vi "Post Tolerance edit.vi"(8 "error in (no error)":errorcluster, 10 "Coords":T1, 11 "ZenGage v3.0 UI in":refnum<class "ZenGage v3.0 UI.lvclass">) -> (0 "error out":errorcluster, 3 "ZenGage v3.0 UI out":refnum<class "ZenGage v3.0 UI.lvclass">)   [LabVIEW 2015, in "ZenGage v3.0 UI.lvclass"]
uses:
  ZenGage v3.0 UI.lvclass
  <vilib>/Utility/miscctls.llb/LVPoint32TypeDef.ctl
  ZenGage v3.0 UI.lvclass/ZenGage v3.0 UI.ctl
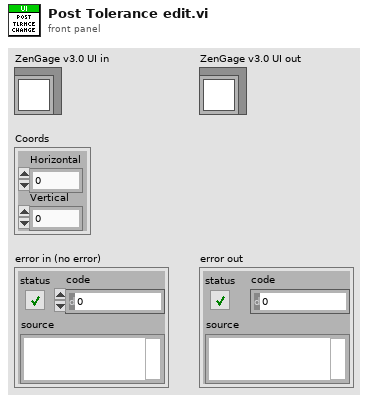
[diagram p1: front panel]
types:
  T1 = typedef "LVPoint32TypeDef.ctl" = cluster{"Horizontal":i32, "Vertical":i32}
  T2 = typedef "ZenGage v3.0 UI.lvclass/Edit Tolerance Input.ctl" = cluster{"ETL controls":T3, "Input Data Cluster":cluster{"Measurement Values":string[][], "Cluster of Limits":cluster{"LSL":dbl, "USL":dbl, "LCL":dbl, "UCL":dbl}, "Rack Selection":T4, "M and N Array":cluster{"M1":u64, "M2":u64, "N1":u64, "N2":u64}[], "Ticked Measurement Index":u32[], "Measurements Enabled":bool[], "Current Active Position":T1, "Current ticked measurement":dbl}}
  T3 = typedef "ETL controls.ctl" = cluster{"Measurement\n ListBox":refnum<vi>, "Cluster of limits":refnum<vi>, "Thresholds limits":refnum<vi>, "Bias Correction":refnum<vi>, "Linearity Correction":refnum<vi>}
  T4 = typedef "ZenGage v3.0 UI.lvclass/Rack Selection.ctl" = enum16{"Both Racks", "Rack 2", "Rack 1"}
  T5 = enum8{"Enabled", "Disabled", "Disabled and Grayed Out"}
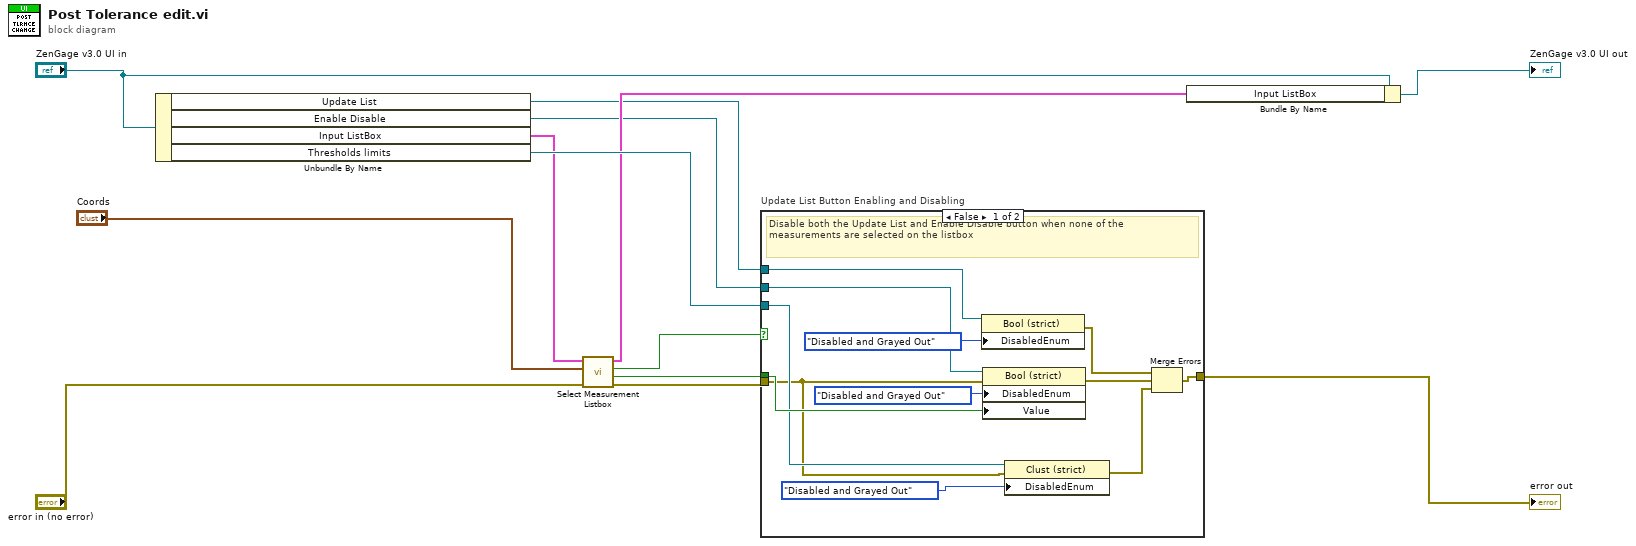
[diagram p0: block diagram]
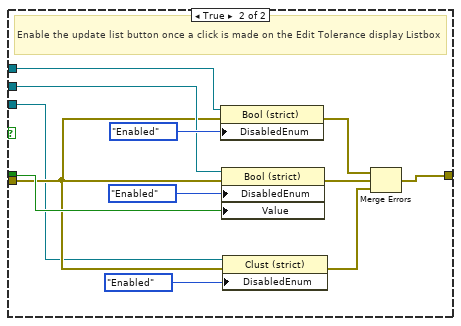
[diagram p2: hidden frame]
diagram:
  n1 = Unbundle By Name("ZenGage v3.0 UI in") -> ("Update List"=w3:refnum<vi>, "Enable Disable"=w4:refnum<vi>, "Input ListBox"=w8:T2, "Thresholds limits"=w12:refnum<vi>)
  n2 = call "Select Measurement Listbox.vi"("error in (no error)"="error in (no error)", "Coords"="Coords", "Input ListBox in"=w8) -> ("error out"=w2:errorcluster, "Enable Disable button state"=w6:bool, "Tick Marked?"=w5:bool, "ListBox Cluster out"=w10:T2)  [unwired: 5 in]
  n3 = case "Update List Button Enabling and Disabling" shown="False" w5 {
    tunnel: w3 -> [w25 w37]
    tunnel: [w20 w32] -> w7
    tunnel: w6 -> [w19 w31]
    tunnel: w2 -> [w16 w29]
    tunnel: w4 -> [w18 w30]
    tunnel: w12 -> [w17 w27]
    frame False {
      # "Disable both the Update List and Enable Disable button when none of the measurements are selected on the listbox"
      n4 = property class="Bool (strict)"(reference=w25, "DisabledEnum"=T5."Disabled and Grayed Out" ("Disabled")) -> (error out=w21:errorcluster)  [unwired: 1 in, 1 out]
      n5 = property class="Bool (strict)"(reference=w18, error in=w16, "DisabledEnum"=T5."Disabled and Grayed Out" ("Disabled"), "Value"=w19) -> (error out=w22:errorcluster)  [unwired: 1 out]
      n6 = property class="Clust (strict)"(reference=w17, error in=w16, "DisabledEnum"=T5."Disabled and Grayed Out" ("Disabled")) -> (error out=w15:errorcluster)  [unwired: 1 out]
      n7 = Merge Errors(w21, w22, w15) -> (w20:errorcluster)
    }
    frame True {
      # "Enable the update list button once a click is made on the Edit Tolerance display Listbox"
      n8 = property class="Bool (strict)"(reference=w37, error in=w29, "DisabledEnum"=T5."Enabled" ("Disabled")) -> (error out=w33:errorcluster)  [unwired: 1 out]
      n9 = property class="Bool (strict)"(reference=w30, error in=w29, "DisabledEnum"=T5."Enabled" ("Disabled"), "Value"=w31) -> (error out=w34:errorcluster)  [unwired: 1 out]
      n10 = property class="Clust (strict)"(reference=w27, error in=w29, "DisabledEnum"=T5."Enabled" ("Disabled")) -> (error out=w28:errorcluster)  [unwired: 1 out]
      n11 = Merge Errors(w33, w34, w28) -> (w32:errorcluster)
    }
  }
  "error out" <- w7
  n12 = Bundle By Name(cluster="ZenGage v3.0 UI in", "Input ListBox"=w10) -> (→"ZenGage v3.0 UI out":refnum<class "ZenGage v3.0 UI.lvclass">)
